vi "Create Filenames.vi"(7 "Format string":string, 8 "Error In":errorcluster, 9 "File name suffixes":string[](array[string]), 10 "Index":i32=-1, 11 "Folder Path Control":path) -> (0 "Error Out":errorcluster, 3 "Paths":path[](array[path]))   [LabVIEW 2024]
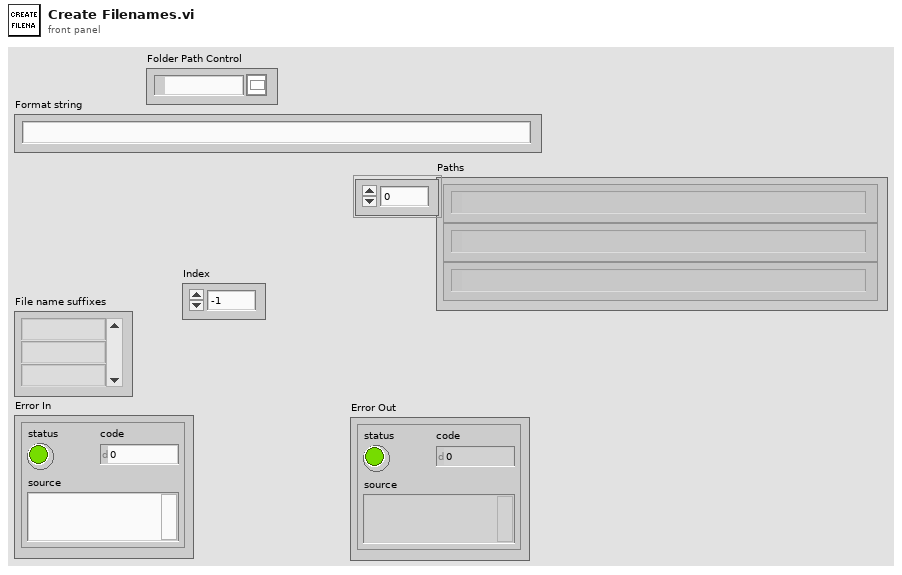
[diagram p1: front panel]
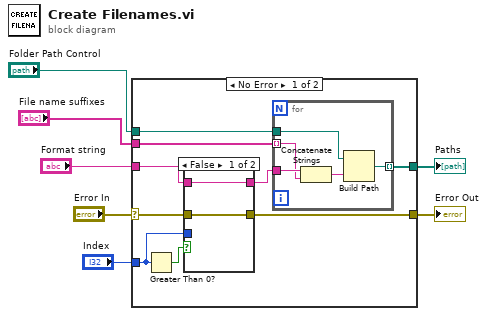
[diagram p0: block diagram]
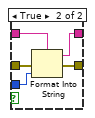
[diagram p2: hidden frame]
diagram:
  n1 = case shown="No Error" "Error In" {
    selector: "Error In" -> [w16 w29]
    tunnel: [w8 w29] -> w6
    tunnel: "Index" -> [w10 _]
    tunnel: "Folder Path Control" -> [w15 _]
    tunnel: [w14 _] -> w3
    tunnel: "File name suffixes" -> [w13 _]
    tunnel: "Format string" -> [w11 _]
    frame No Error {
      n2 = Greater Than 0?(x=w10) -> (x > 0?=w9:bool)
      n3 = case shown="False" w9 {
        tunnel: w16 -> [w18 w23]
        tunnel: [w17 w22] -> w12
        tunnel: [w18 w21] -> w8
        tunnel: w11 -> [w17 w20]
        tunnel: w10 -> [_ w19]
        frame False {
        }
        frame True {
          n4 = Format Into String(format string=w20, error in=w23, w19) -> (resulting string=w22:string, error out=w21:errorcluster)  [unwired: 1 in]
        }
      }
      n5 = for {
        tunnel: w12 -> [w28]
        tunnel: [w24] -> w14 mode=indexing
        tunnel: w13 -> [w27] mode=indexing
        tunnel: w15 -> [w26]
        n6 = Concatenate Strings(w28, w27) -> (w25:string)
        n7 = Build Path(base path=w26, name or relative path=w25) -> (appended path=w24:path)
      }
    }
    frame Error {
    }
  }
  "Error Out" <- w6
  "Paths" <- w3
